vi "ListClassItems.vi"(8 "error in (no error)":errorcluster, 9 "Return references (F)":bool, 11 "LVClass refnum":refnum<vi>) -> (0 "error out":errorcluster, 1 "ItemReferences":refnum<vi>[](array[refnum]), 2 "Class Items":string[](array[string]), 3 "dup LVClass refnum":refnum<vi>)   [LabVIEW 2019, in "BlueUtilityScripts.lvlib"]
uses:
  BlueUtilityScripts.lvlib
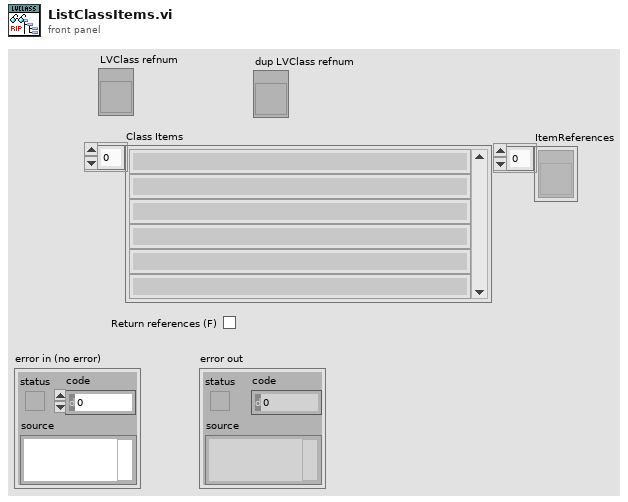
[diagram p1: front panel]
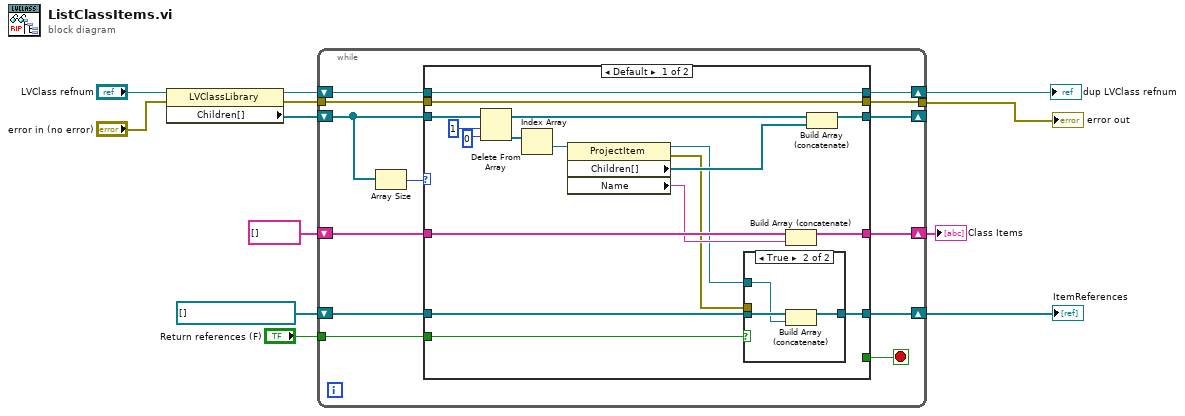
[diagram p0: block diagram]
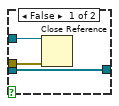
[diagram p2: hidden frame]
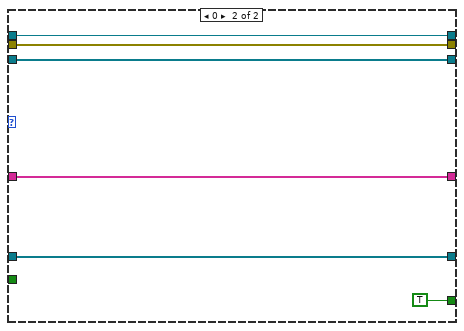
[diagram p3: hidden frame]
diagram:
  n1 = property class="LVClassLibrary"(reference="LVClass refnum", error in="error in (no error)") -> (reference out=w11:refnum<vi>, error out=w5:errorcluster, "Children[]"=w10:refnum<vi>[])
  n2 = while {
    shift-right: [w22] -> _
    shift-left: w10 -> [w23]
    shift-right: [w20] -> w8
    shift-left: string[] [] -> [w21]
    tunnel: w5 -> [w17]
    tunnel: [w16] -> w4
    shift-right: [w13] -> w1
    shift-left: refnum<vi>[] [] -> [w15]
    tunnel: "Return references (F)" -> [w14]
    shift-right: [w18] -> w6
    shift-left: w11 -> [w19]
    stop <- w24 stop-if-true
    n3 = Array Size(array=w23) -> (size(s)=w25:i32)
    n4 = case shown="Default" w25 {
      tunnel: [_ TRUE] -> w24
      tunnel: w23 -> [w42 w54]
      tunnel: [w36 w54] -> w22
      tunnel: w21 -> [w35 w53]
      tunnel: [w33 w53] -> w20
      tunnel: w19 -> [w32 w52]
      tunnel: [w32 w52] -> w18
      tunnel: w17 -> [w31 w51]
      tunnel: [w31 w51] -> w16
      tunnel: w15 -> [w30 w50]
      tunnel: w14 -> [w28 _]
      tunnel: [w29 w50] -> w13
      frame Default {
        n5 = Delete From Array(array=w42, length=1 ("Length"), index=0 ("Length")) -> (deleted portion=w40:refnum<vi>[], array with subset deleted=w38:refnum<vi>[])
        n6 = Index Array(array=w40) -> (element=w39:refnum<vi>)  [unwired: 1 in]
        n7 = property class="ProjectItem"(reference=w39) -> (reference out=w27:refnum<vi>, error out=w26:errorcluster, "Children[]"=w37:refnum<vi>[], "Name"=w34:string)  [unwired: 1 in]
        n8 = case shown="True" w28 {
          tunnel: w30 -> [w46 w49]
          tunnel: [w46 w48] -> w29
          tunnel: w27 -> [w45 w47]
          tunnel: w26 -> [w44 _]
          frame False {
            n9 = Close Reference(reference=w45, error in (no error)=w44) -> ()  [unwired: 1 out]
          }
          frame True {
            n10 = Build Array (concatenate)(w49, w47) -> (w48:refnum<vi>[])
          }
        }
        n11 = Build Array (concatenate)(w35, w34) -> (w33:string[])
        n12 = Build Array (concatenate)(w38, w37) -> (w36:refnum<vi>[])
      }
      frame 0 {
      }
    }
  }
  "error out" <- w4
  "dup LVClass refnum" <- w6
  "Class Items" <- w8
  "ItemReferences" <- w1
